vi "Disconnect Terminals.vi"(8 "error in (no error)":errorcluster, 11 "CRDS in":refnum<class "CRDS.lvclass">) -> (0 "error out":errorcluster, 3 "CRDS out":refnum<class "CRDS.lvclass">)   [LabVIEW 2011, in "CRDS.lvclass"]
uses:
  CRDS.lvclass
  CRDS.lvclass/CRDS.ctl
  Program Files/National Instruments/LabVIEW 2011/resource/objmgr/daqmx.rc
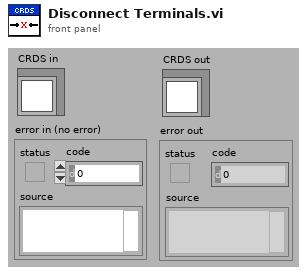
[diagram p1: front panel]
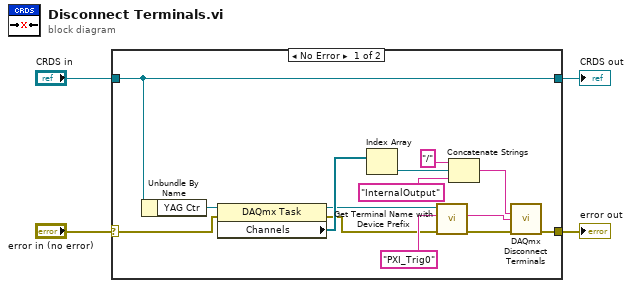
[diagram p0: block diagram]
diagram:
  n1 = case shown="No Error" "error in (no error)" {
    selector: "error in (no error)" -> [w6 w20]
    tunnel: [w8 w20] -> w3
    tunnel: [w9 w19] -> w1
    tunnel: "CRDS in" -> [w9 w19]
    frame No Error {
      n2 = Unbundle By Name(w9) -> ("YAG Ctr"=w16:refnum<k21>)
      n3 = property class="DAQmx Task"(reference=w16, error in=w6) -> (reference out=w7:refnum<k21>, error out=w5:errorcluster, "Channels"=w17:refnum<k21>[])
      n4 = Index Array(array=w17) -> (element=w18:refnum<k21>)  [unwired: 1 in]
      n5 = call "Get Terminal Name with Device Prefix.vi"("error in (no error)"=w5, "Local Terminal Name"="PXI_Trig0", "task/channels in"=w7) -> ("error out"=w13:errorcluster, "Terminal Name with Device Prefix"=w11:tag)  [unwired: 6 in, 1 out]
      n6 = Concatenate Strings("/", w18, "InternalOutput" ("string")) -> (w10:string)
      n7 = call <vilib>:"DAQmx Disconnect Terminals.vi"("source terminal"=w10, "destination terminal"=w11, "error in"=w13) -> ("error out"=w8:errorcluster)  [unwired: 12 in]
    }
    frame Error {
    }
  }
  "error out" <- w3
  "CRDS out" <- w1
